vi "Command No-Op.vi"(7 "Startup":bool) -> (4 "Reint":bool, 6 "Completed":bool)   [LabVIEW 2018]
uses:
  Autonomous Utilities/Command_Execution_State.ctl
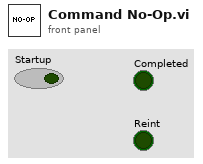
[diagram p1: front panel]
types:
  T1 = typedef "Command_Execution_State.ctl" = enum16{"Initialize", "Execute", "Finish"}
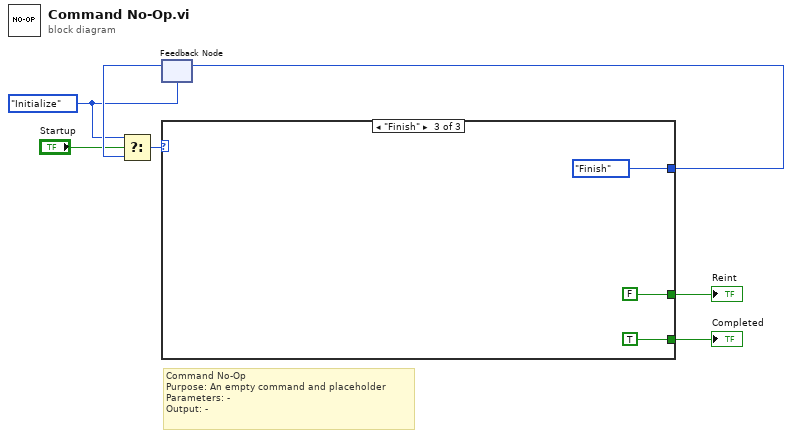
[diagram p0: block diagram]
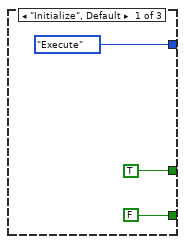
[diagram p2: hidden frame]
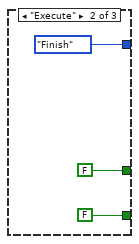
[diagram p3: hidden frame]
diagram:
  w1 = Command_Execution_State."Initialize" ("Play State")
  # "Command No-Op\nPurpose: An empty command and placeholder\nParameters: -\nOutput: -"
  n1 = feedback #1(w1) -> (w5:T1)
  n2 = Select(t=w1, s="Startup", f=w5) -> (s? t:f=w7:T1)
  n3 = case shown="\"Finish\"" w7 {
    tunnel: [Command_Execution_State."Execute" ("Play State") Command_Execution_State."Finish" ("Play State") Command_Execution_State."Finish" ("Play State")] -> w6
    tunnel: [FALSE FALSE TRUE] -> w4
    tunnel: [TRUE FALSE FALSE] -> w2
    frame "Initialize", Default {
    }
    frame "Execute" {
    }
    frame "Finish" {
    }
  }
  "Completed" <- w4
  "Reint" <- w2
  n4 = feedback-in #1(w6) -> ()
